vi "B&KCorrect.vi"(0 "sample rate MHz":u16, 1 "attenuation (dB/MHz/cm)":dbl=0.5 format="%.2f", 2 "Fit params":T1 {"pts in fit" format="%.2f"; "midband fit" format="%.2f"; "intercept (b)" format="%.2f"; "slope (m)" format="%.2f"}, 3 "Fit band":cluster{dbl, "stop freq":dbl, "center freq":dbl} {"center freq" format="%.2f"; "stop freq" format="%.2f"; "?" format="%.2f"}, 4 "Array Subset":T2) -> (6 "Fit params Corrected":T1 {"pts in fit" format="%.2f"; "midband fit" format="%.2f"; "intercept (b)" format="%.2f"; "slope (m)" format="%.2f"})   [LabVIEW 2022 SP3]
panel:
  out "MB correction":dbl format="%.2f"
  out "window correction":dbl format="%.4f"
  out "slope correction":dbl format="%.2f"
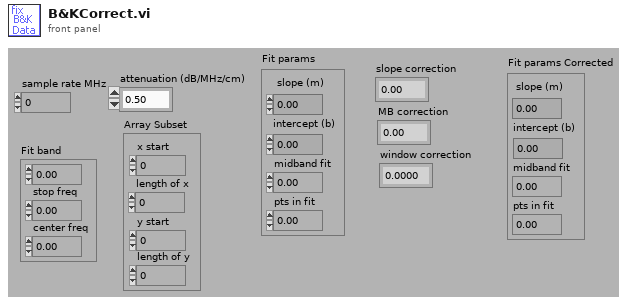
[diagram p1: front panel]
types:
  T1 = cluster{"slope (m)":dbl, "intercept (b)":dbl, "midband fit":dbl, "pts in fit":dbl}
  T2 = cluster{"x start":i32, "length of x":i32, "y start":i32, "length of y":i32}
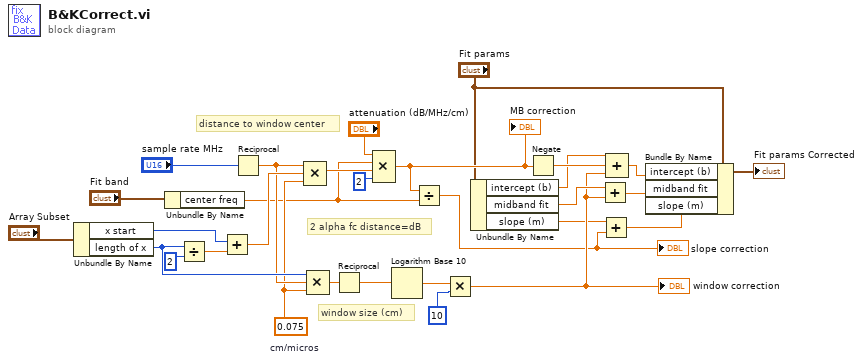
[diagram p0: block diagram]
diagram:
  w23 = 0.075  # cm/micros
  # "2 alpha fc distance=dB"
  # "distance to window center"
  # "window size (cm)"
  n1 = Unbundle By Name("Array Subset") -> ("x start"=w27:i32, "length of x"=w25:i32)
  n2 = Unbundle By Name("Fit band") -> ("center freq"=w3:dbl)
  n3 = Divide(x=w25, y=2) -> (x/y=w28:dbl)
  n4 = Add(x=w27, y=w28) -> (x+y=w26:dbl)
  n5 = Reciprocal(x="sample rate MHz") -> (1/x=w24:dbl)
  n6 = Compound Arithmetic op=MULTIPLY(w24, w26, w23) -> (w16:dbl)
  n7 = Compound Arithmetic op=MULTIPLY(w25, w24, w23) -> (w22:dbl)
  n8 = Reciprocal(x=w22) -> (1/x=w18:dbl)
  n9 = Compound Arithmetic op=MULTIPLY("attenuation (dB/MHz/cm)", w3, w16, 2) -> (w13:dbl)
  "MB correction" <- w13
  n10 = Logarithm Base 10(1:w18) -> (0:w21:dbl)
  n11 = Divide(x=w13, y=w3) -> (x/y=w8:dbl)
  "slope correction" <- w8
  n12 = Multiply(x=w21, y=10) -> (x*y=w11:dbl)
  "window correction" <- w11
  n13 = Unbundle By Name("Fit params") -> ("intercept (b)"=w10:dbl, "midband fit"=w14:dbl, "slope (m)"=w9:dbl)
  n14 = Negate(x=w13) -> (-x=w12:dbl)
  n15 = Add(x=w14, y=w11) -> (x+y=w1:dbl)
  n16 = Add(x=w9, y=w8) -> (x+y=w6:dbl)
  n17 = Compound Arithmetic op=ADD(w10, w12, w11) -> (w2:dbl)
  n18 = Bundle By Name(cluster="Fit params", "intercept (b)"=w2, "midband fit"=w1, "slope (m)"=w6) -> (→"Fit params Corrected":T1)
